vi "DSF.Engine.Interface.Destroy.vi"(8 "error in (no error)":errorcluster, 11 "Interface in":refnum<class "DSF.Engine.Interface.lvclass">) -> (0 "error out":errorcluster, 2 "remaining errors":errorcluster[](array[cluster]), 3 "Interface out":refnum<class "DSF.Engine.Interface.lvclass">)   [LabVIEW 2017, in "Data Sharing Framework Engine.lvlib" / "DSF.Engine.Interface.lvclass"]
uses:
  DSF.Engine.Interface.lvclass
  DSF.Engine.Interface.lvclass/DSF.Engine.Interface.ctl
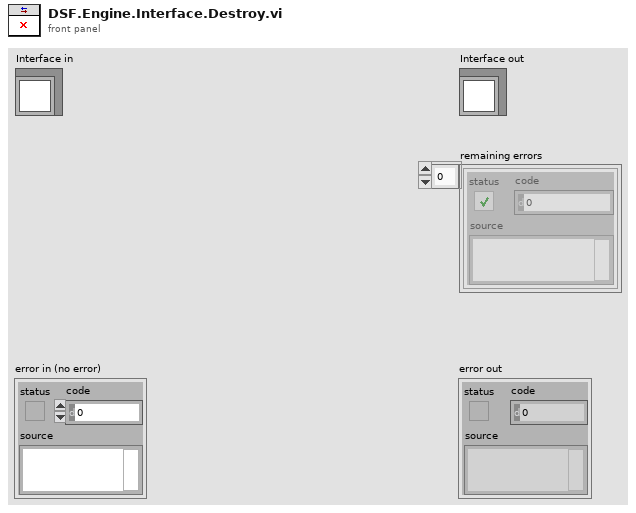
[diagram p1: front panel]
types:
  T1 = typedef "Data Sharing Framework Engine.lvlib/DSF.Engine.Interface.lvclass/DSF.Engine.Interface.RT FIFO.Ref.16B.ctl" = refnum<k33>
  T2 = typedef "Data Sharing Framework Engine.lvlib/DSF.Engine.Interface.lvclass/DSF.Engine.Interface.Error Queue.Ref.ctl" = refnum<queue>
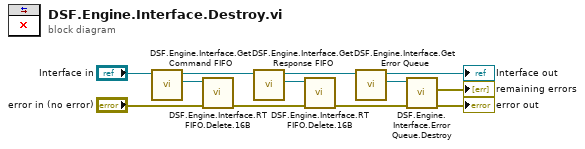
[diagram p0: block diagram]
diagram:
  n1 = call "DSF.Engine.Interface.Get Command FIFO.vi"("Interface in"="Interface in") -> ("Command FIFO"=w10:T1, "Interface out"=w11:refnum<class "DSF.Engine.Interface.lvclass">)  [unwired: 9 in]
  n2 = call "DSF.Engine.Interface.RT FIFO.Delete.16B.vi"("error in (no error)"="error in (no error)", "RT FIFO"=w10) -> ("error out"=w7:errorcluster)  [unwired: 9 in]
  n3 = call "DSF.Engine.Interface.Get Response FIFO.vi"("Interface in"=w11) -> ("Response FIFO"=w9:T1, "Interface out"=w6:refnum<class "DSF.Engine.Interface.lvclass">)  [unwired: 9 in]
  n4 = call "DSF.Engine.Interface.RT FIFO.Delete.16B.vi"("error in (no error)"=w7, "RT FIFO"=w9) -> ("error out"=w4:errorcluster)  [unwired: 9 in]
  n5 = call "DSF.Engine.Interface.Get Error Queue.vi"("Interface in"=w6) -> ("Error Queue"=w5:T2, "Interface out"=→"Interface out":refnum<class "DSF.Engine.Interface.lvclass">)  [unwired: 9 in]
  n6 = call "DSF.Engine.Interface.Error Queue.Destroy.vi"("error in (no error)"=w4, "Error Queue"=w5) -> ("error out"=→"error out":errorcluster, "remaining errors"=→"remaining errors":errorcluster[])  [unwired: 8 in]
